vi "DB Action Engine SubVI.vi"(2 "Connection Information":string[](array[string]), 7 "Cmd":T1, 8 "error in (no error)":errorcluster, 10 "MySQL Credentials":T3={"Server"="EXELIQ", " User ID"="EXELIQ", "Password"="Exeliq2617"}, 11 "Query String":string) -> (0 "error out":errorcluster, 1 "data":variant[][](array[variant]), 3 "connection reference":T2)   [LabVIEW 2021]
uses:
  Controls/MySQL Credential Control.ctl
  <vilib>/addons/database/Connection.llb/Conn ObjectReference.ctl
  Controls/Enum.ctl
  <vilib>/addons/database/Auxilliary.llb/DB Tools Cursor Type.ctl
  <vilib>/addons/database/Connection.llb/DB Tools Open Connec (String).vi
  <vilib>/addons/database/Connection.llb/Conn Execute.vi
  <vilib>/addons/database/Recordset.llb/Rec Fetch Recordset Data (R).vi
  <vilib>/addons/database/Recordset.llb/Rec Destroy - Connection.vi
  <vilib>/addons/database/NI_Database_API.lvlib
panel:
  out "Resulting string":string
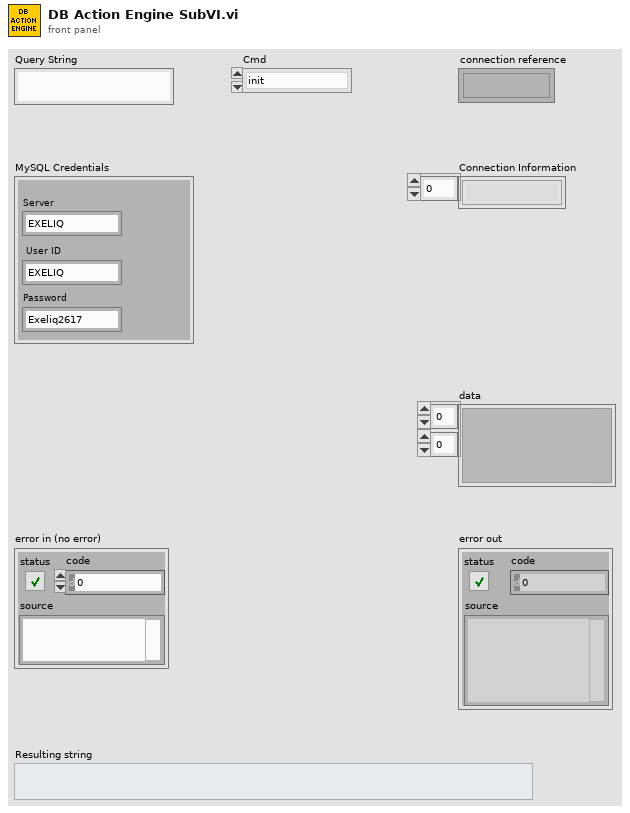
[diagram p1: front panel]
types:
  T1 = typedef "Enum.ctl" = enum16{"init", "Execute Query", "Close"}
  T2 = typedef "NI_Database_API.lvlib/Conn ObjectReference.ctl" = refnum<k1>
  T3 = typedef "MySQL Credential Control.ctl" = cluster{"Server":string, " User ID":string, "Password":string}
  T4 = typedef "NI_Database_API.lvlib/DB Tools Cursor Type.ctl" = enum16{"forward-only", "keyset", "dynamic", "static"}
  T5 = typedef "NI_Database_API.lvlib/Rec ObjectReference.ctl" = refnum<k1>
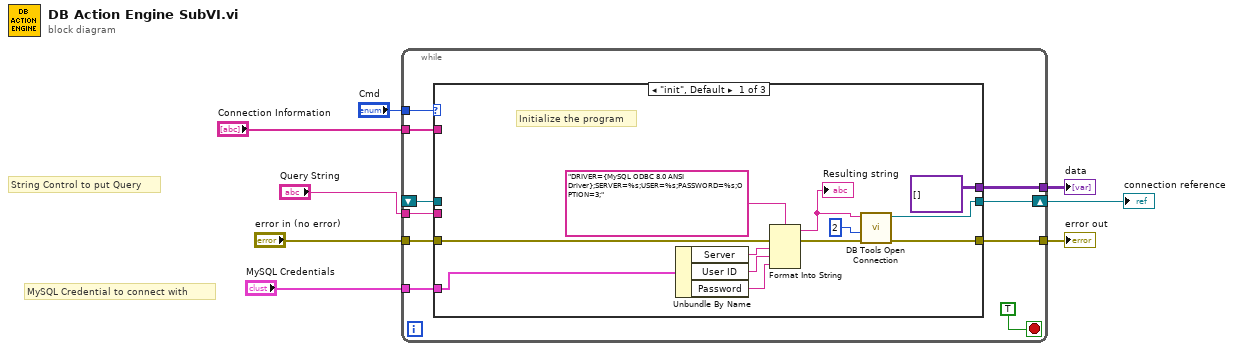
[diagram p0: block diagram]
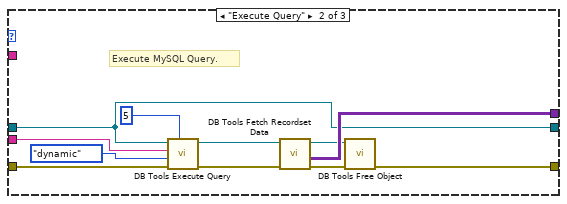
[diagram p2: hidden frame]
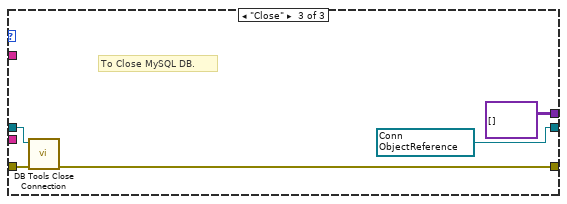
[diagram p3: hidden frame]
diagram:
  # "MySQL Credential to connect with"
  # "String Control to put Query"
  n1 = while {
    tunnel: "error in (no error)" -> [w18]
    tunnel: [w17] -> w7
    tunnel: "Connection Information" -> [w16]
    shift-right: [w15] -> w2
    shift-left: _ -> [w13]
    tunnel: "Query String" -> [w14]
    tunnel: [w11] -> w4
    tunnel: "Cmd" -> [w10]
    tunnel: "MySQL Credentials" -> [w9]
    stop <- TRUE stop-if-true
    n2 = case shown="\"init\", Default" w10 {
      tunnel: w18 -> [w26 w41 w46]
      tunnel: [w24 w33 w45] -> w17
      tunnel: w16 -> [_ _ _]
      tunnel: [w25 w31 w43] -> w15
      tunnel: w14 -> [_ w40 _]
      tunnel: w13 -> [_ w31 w44]
      tunnel: [variant[][] [] ("data") w35 variant[][] [] ("data")] -> w11
      tunnel: w9 -> [w22 _ _]
      frame "init", Default {
        # "Initialize the program"
        n3 = Unbundle By Name(w22) -> ("Server"=w21:string, "User ID"=w20:string, "Password"=w19:string)
        n4 = Format Into String(format string="DRIVER={MySQL ODBC 8.0 ANSI Driver};SERVER=%s;USER=%s;PASSWORD=%s;OPTION=3;", error in=w26, w21, w20, w19) -> (resulting string=w23:string, error out=w29:errorcluster)  [unwired: 1 in]
        "Resulting string" <- w23
        n5 = call-poly <vilib>:"DB Tools Open Connection.vi"("error in (no error)"=w29, "connection timeout (15)"=2, "connection information"=w23) -> ("error out"=w24:errorcluster, "connection reference"=w25:T2)  [unwired: 5 in]
      }
      frame "Execute Query" {
        # "Execute MySQL Query."
        n6 = call-poly <vilib>:"DB Tools Execute Query.vi"("cache size (1)"=5, "error in (no error)"=w41, "cursor type"=DB_Tools_Cursor_Type."dynamic", "SQL query"=w40, "connection reference"=w31) -> ("error out"=w36:errorcluster, "recordset reference"=w37:T5)  [unwired: 3 in]
        n7 = call-poly <vilib>:"DB Tools Fetch Recordset Data.vi"("error in (no error)"=w36, "recordset reference"=w37) -> ("error out"=w34:errorcluster, "recordset data"=w35:variant[][], "recordset reference out"=w32:T5)  [unwired: 3 in]
        n8 = call-poly <vilib>:"DB Tools Free Object.vi"("error in (no error)"=w34, "recordset reference"=w32) -> ("error out"=w33:errorcluster)  [unwired: 8 in, 1 out]
      }
      frame "Close" {
        w43 = T2 refnum items=["Connection"] ("connection reference")
        # "To Close MySQL DB."
        n9 = call <vilib>:"DB Tools Close Connection.vi"("error in (no error)"=w46, "connection reference"=w44) -> ("error out"=w45:errorcluster)  [unwired: 5 in]
      }
    }
  }
  "error out" <- w7
  "data" <- w4
  "connection reference" <- w2
